vi "another-array.vi"() -> ()   [LabVIEW 2025]
panel:
  in  "Array 4":dbl[](array[numeric])
  out "Numeric 3":dbl
  in  "Numeric 2":dbl
  out "Numeric":dbl
  out "Array 2":dbl[](array[numeric])
  out "Array 3":dbl[](array[numeric])
  in  "Array":dbl[](array[numeric])
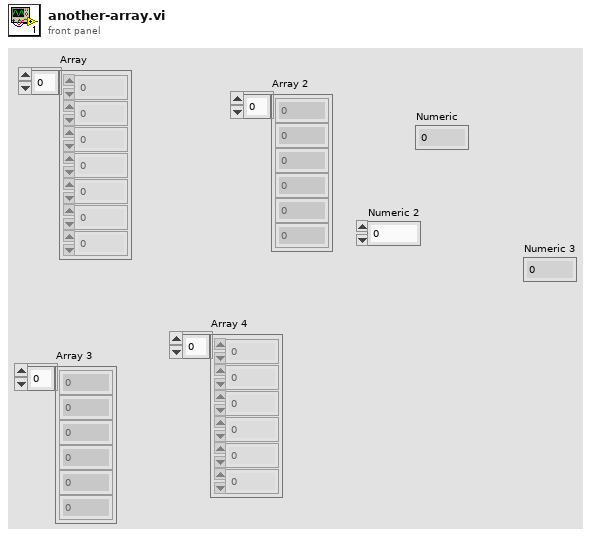
[diagram p1: front panel]
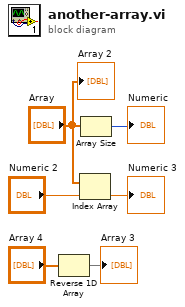
[diagram p0: block diagram]
diagram:
  n1 = Reverse 1D Array(array="Array 4") -> (reversed array=→"Array 3":dbl[])
  n2 = Index Array(array="Array", index="Numeric 2") -> (element=→"Numeric 3":dbl)
  n3 = Array Size(array="Array") -> (size(s)=→"Numeric":i32)
  "Array 2" <- "Array"
